vi "XYStage.ConvertScalar.vi"(8 "error in (no error)":errorcluster, 9 "Counts":i32, 10 "Units":dbl, 11 "XYStage in":refnum<class "XYStage.lvclass">) -> (0 "error out":errorcluster, 1 "Units out":dbl, 2 "Counts out":i32, 3 "XYStage out":refnum<class "XYStage.lvclass">)   [LabVIEW 2015, in "XYStage.lvclass"]
uses:
  XYStage.lvclass
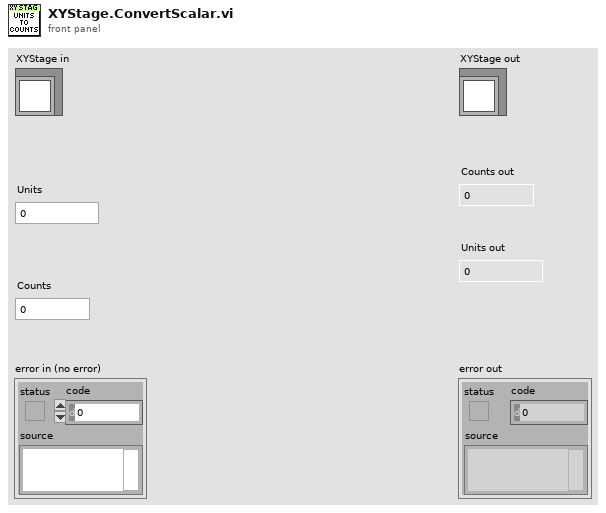
[diagram p1: front panel]
types:
  T1 = typedef "XYStage.lvclass/Configuration--Cluster.ctl" = cluster{"Real-World Units":string, "Counts per Unit":dbl}
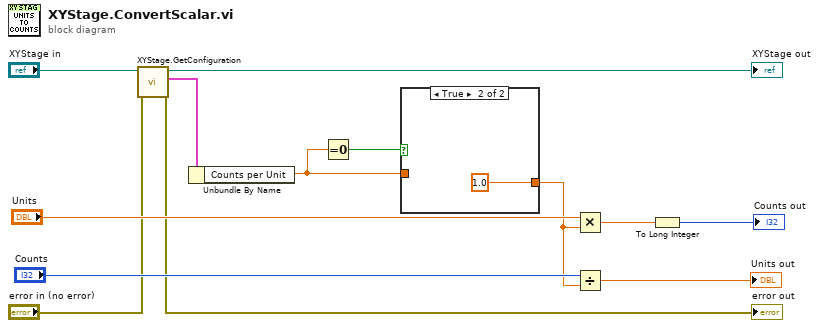
[diagram p0: block diagram]
diagram:
  n1 = call "XYStage.GetConfiguration.vi"("error in (no error)"="error in (no error)", "XYStage"="XYStage in") -> ("error out"=→"error out":errorcluster, "Configuration"=w4:T1, "XYStage out"=→"XYStage out":refnum<class "XYStage.lvclass">)  [unwired: 7 in]
  n2 = Unbundle By Name(w4) -> ("Counts per Unit"=w3:dbl)
  n3 = Equal To 0?(x=w3) -> (x = 0?=w2:bool)
  n4 = case shown="True" w2 {
    tunnel: [w14 1.0 ("X")] -> w5
    tunnel: w3 -> [w14 _]
    frame False {
    }
    frame True {
    }
  }
  n5 = Multiply(x="Units", y=w5) -> (x*y=w12:dbl)
  n6 = Divide(x="Counts", y=w5) -> (x/y=→"Units out":dbl)
  n7 = To Long Integer(number=w12) -> (32bit integer=→"Counts out":i32)
